vi "Get IPF folder.vi"(8 "error in (no error)":errorcluster) -> (0 "error out":errorcluster, 1 "Results Folder":path, 2 "IPF sub folders":path[](array[path]), 3 "IPF Folder":path, 4 "program names":string[](array[string]), 5 "Results sub folders":path[](array[path]))   [LabVIEW 2013, in "Manipulate IPF.lvlib"]
uses:
  Manipulate IPF.lvlib
  <vilib>/Utility/sysdir.llb/System Directory Type.ctl
  <userlib>/_OpenG.lib/file/file.llb/Strip Path Extension - 1D Array of Strings__ogtk.vi
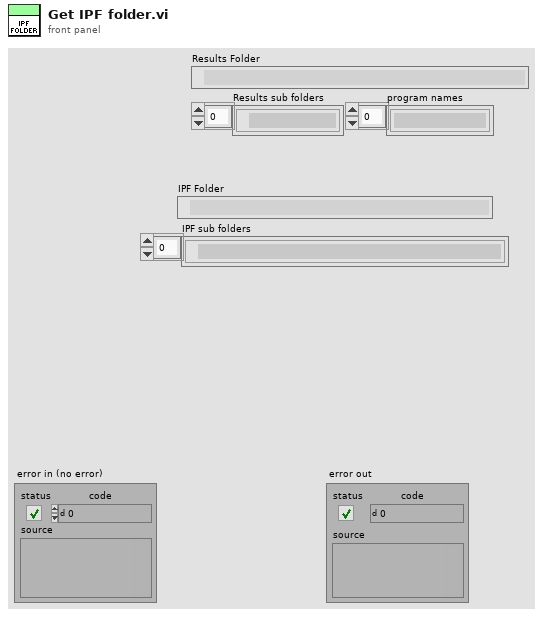
[diagram p1: front panel]
types:
  T1 = typedef "System Directory Type.ctl" = i32
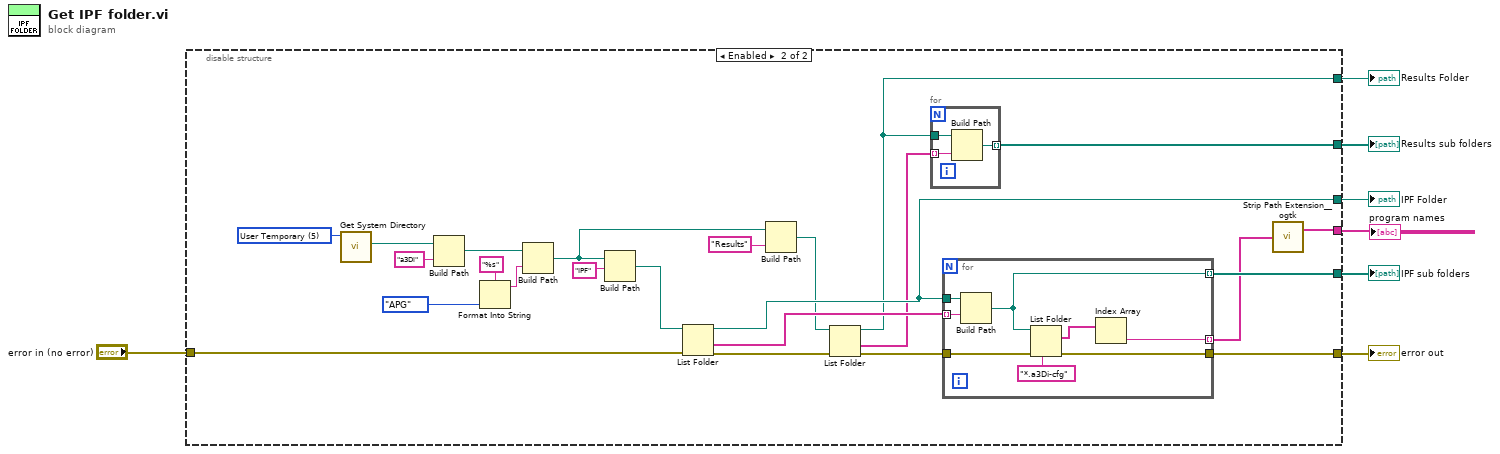
[diagram p0: block diagram]
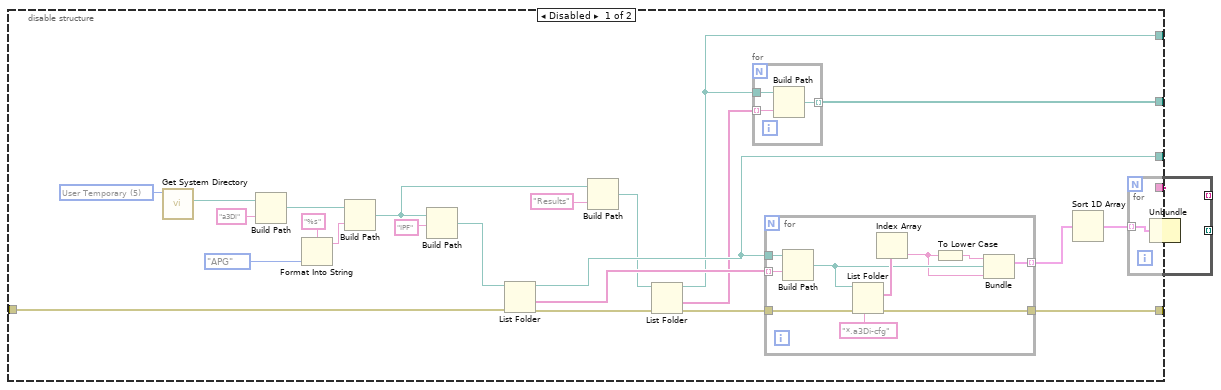
[diagram p2: hidden frame]
diagram:
  n1 = disable-structure shown="Enabled" {
    disable-tunnel: [w23 w63] -> w7
    disable-tunnel: "error in (no error)" -> [w22 w62]
    disable-tunnel: [w19 w59] -> w5
    disable-tunnel: [w18 w58] -> w4
    disable-tunnel: [w12 w52] -> w3
    disable-tunnel: [w10 w53] -> w2
    disable-tunnel: [w9 w51] -> w1
    frame Disabled {
      w33 = T1 5 items=["User Home"=0, "User Desktop"=1, "User Documents"=2, "User Application Data"=3, "User Preferences"=4, "User Temporary"=5, "Public Documents"=6, "Public Application Data"=7, "Public Preferences"=8, "Public Cache"=13, "System Core Libraries"=9, "System Installed Libraries"=10, "Application Files"=11, "Boot Volume Root"=12] ("system directory type")
      n2 = call <vilib>:"Get System Directory.vi"("system directory type"=w33) -> ("system directory"=w32:path)  [unwired: 10 in]
      n3 = Build Path(base path=w32, name or relative path="a3Di") -> (appended path=w31:path)
      n4 = Format Into String(format string="%s", enum16{"APG", "Inspection", "Diagnostic"}."APG" ("a3Di Stations")) -> (resulting string=w29:string)  [unwired: 2 in, 1 out]
      n5 = Build Path(base path=w31, name or relative path=w29) -> (appended path=w15:path)
      n6 = Build Path(base path=w15, name or relative path="IPF") -> (appended path=w25:path)
      n7 = List Folder(path=w25, error in=w22) -> (path out=w23:path, folder names=w24:string[], error out=w16:errorcluster)  [unwired: 2 in, 1 out]
      n8 = Build Path(base path=w15, name or relative path="Results") -> (appended path=w20:path)
      n9 = List Folder(path=w20, error in=w16) -> (path out=w19:path, folder names=w17:string[], error out=w11:errorcluster)  [unwired: 2 in, 1 out]
      n10 = for {
        tunnel: w19 -> [w39]
        tunnel: [w38] -> w18 mode=indexing
        tunnel: w17 -> [w37] mode=indexing
        n11 = Build Path(base path=w39, name or relative path=w37) -> (appended path=w38:path)
      }
      n12 = for {
        tunnel: w24 -> [w49] mode=indexing
        tunnel: w23 -> [w48]
        tunnel: [w45] -> w14 mode=indexing
        tunnel: w11 -> [w44]
        tunnel: [w43] -> w10
        n13 = Build Path(base path=w48, name or relative path=w49) -> (appended path=w46:path)
        n14 = List Folder(path=w46, pattern="*.a3Di-cfg", error in=w44) -> (filenames=w47:string[], error out=w43:errorcluster)  [unwired: 1 in, 2 out]
        n15 = Index Array(array=w47) -> (element=w41:string)  [unwired: 1 in]
        n16 = To Lower Case(string=w41) -> (all lower case string=w40:string)
        n17 = Bundle(w40, "appended path"=w46, w41) -> (w45:cluster{string, "appended path":path, string})  [unwired: 1 in]
      }
      n18 = Sort 1D Array(array=w14) -> (sorted array=w13:cluster{string, "appended path":path, string}[])
      n19 = for {
        tunnel: w13 -> [w36] mode=indexing
        tunnel: [w35] -> w12 mode=indexing
        tunnel: [w34] -> w8 mode=indexing
        n20 = Unbundle(w36) -> ("appended path"=w35:path, w34:string)  [unwired: 1 out]
      }
      n21 = call-poly <userlib>:"Strip Path Extension__ogtk.vi"("paths"=w8) -> ("roots"=w9:string[])  [unwired: 1 out]
    }
    frame Enabled {
      w73 = T1 5 items=["User Home"=0, "User Desktop"=1, "User Documents"=2, "User Application Data"=3, "User Preferences"=4, "User Temporary"=5, "Public Documents"=6, "Public Application Data"=7, "Public Preferences"=8, "Public Cache"=13, "System Core Libraries"=9, "System Installed Libraries"=10, "Application Files"=11, "Boot Volume Root"=12] ("system directory type")
      n22 = call <vilib>:"Get System Directory.vi"("system directory type"=w73) -> ("system directory"=w72:path)  [unwired: 10 in]
      n23 = Build Path(base path=w72, name or relative path="a3Di") -> (appended path=w71:path)
      n24 = Format Into String(format string="%s", enum16{"APG", "Inspection", "Diagnostic"}."APG" ("a3Di Stations")) -> (resulting string=w69:string)  [unwired: 2 in, 1 out]
      n25 = Build Path(base path=w71, name or relative path=w69) -> (appended path=w55:path)
      n26 = Build Path(base path=w55, name or relative path="IPF") -> (appended path=w65:path)
      n27 = List Folder(path=w65, error in=w62) -> (path out=w63:path, folder names=w64:string[], error out=w56:errorcluster)  [unwired: 2 in, 1 out]
      n28 = Build Path(base path=w55, name or relative path="Results") -> (appended path=w60:path)
      n29 = List Folder(path=w60, error in=w56) -> (path out=w59:path, folder names=w57:string[], error out=w54:errorcluster)  [unwired: 2 in, 1 out]
      n30 = for {
        tunnel: w59 -> [w76]
        tunnel: [w75] -> w58 mode=indexing
        tunnel: w57 -> [w74] mode=indexing
        n31 = Build Path(base path=w76, name or relative path=w74) -> (appended path=w75:path)
      }
      n32 = for {
        tunnel: w64 -> [w84] mode=indexing
        tunnel: w63 -> [w83]
        tunnel: [w78] -> w50 mode=indexing
        tunnel: w54 -> [w81]
        tunnel: [w80] -> w53
        tunnel: [w77] -> w52 mode=indexing
        n33 = Build Path(base path=w83, name or relative path=w84) -> (appended path=w77:path)
        n34 = List Folder(path=w77, pattern="*.a3Di-cfg", error in=w81) -> (filenames=w82:string[], error out=w80:errorcluster)  [unwired: 1 in, 2 out]
        n35 = Index Array(array=w82) -> (element=w78:string)  [unwired: 1 in]
      }
      n36 = call-poly <userlib>:"Strip Path Extension__ogtk.vi"("paths"=w50) -> ("roots"=w51:string[])  [unwired: 1 out]
    }
  }
  "IPF sub folders" <- w3
  "IPF Folder" <- w7
  "error out" <- w2
  "Results Folder" <- w5
  "Results sub folders" <- w4
  "program names" <- w1
